vi "WriteSV.vi"(8 "error in (no error)":errorcluster, 10 "DBL Data":dbl, 11 "shared variable refnum in":refnum<k21>) -> (0 "error out":errorcluster)   [LabVIEW 2016, in "Shared Variable Interface.lvlib" / "DBL.lvlib"]
uses:
  DBL.lvlib
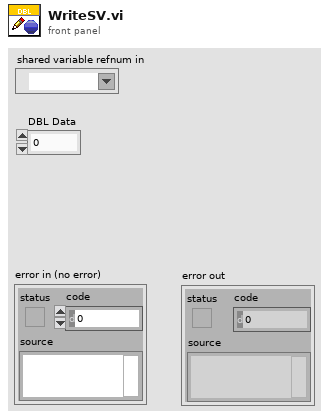
[diagram p1: front panel]
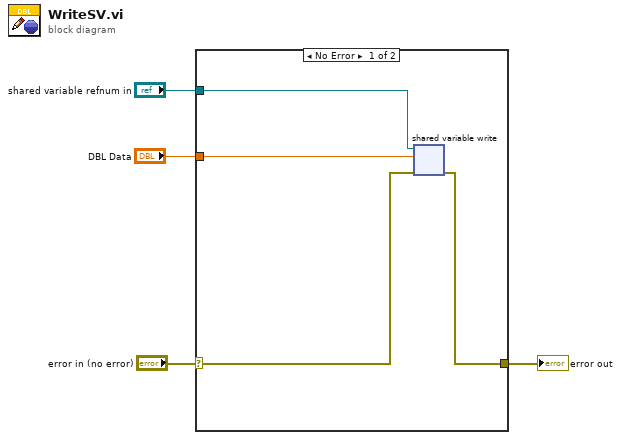
[diagram p0: block diagram]
diagram:
  n1 = case shown="No Error" "error in (no error)" {
    selector: "error in (no error)" -> [w6 w9]
    tunnel: [w8 w9] -> w4
    tunnel: "DBL Data" -> [w7 _]
    tunnel: "shared variable refnum in" -> [w5 _]
    frame No Error {
      n2 = shared-variable-write(w5, w6, w7) -> (w8:errorcluster)  [unwired: 1 out]
    }
    frame Error {
    }
  }
  "error out" <- w4
